vi "AlliGator Init Image Profile Window Menu.vi"(8 "error in":errorcluster, 11 "Menu in":refnum<k9>) -> (0 "error out":errorcluster)   [LabVIEW 2021, in "AlliGator Image Profile Window.lvlib"]
doc: "Initialize Profile Window menu."
uses:
  AlliGator Image Profile Window.lvlib
  Globals, Variables, Constants/AlliGator Variables List.ctl
  Image/Box Profile Type.ctl
  AlliGator Image Profile Intensity Type.ctl
  AlliGator Image Profile Average Intensity Type.ctl
  Globals, Variables, Constants/AlliGator Globals, Variables & Constants.lvlib
  Image/Image.lvlib
panel:
  # "see the AlliGator License on the block diagram (Ctrl+E or Window:Show Block Diagram)"
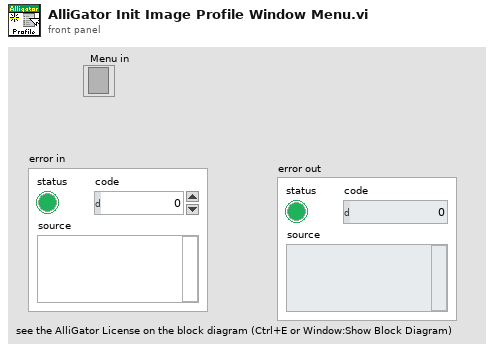
[diagram p1: front panel]
types:
  T1 = typedef "AlliGator Image Profile Window.lvlib/AlliGator Image Profile Average Intensity Type.ctl" = enum16{"Integrated Intensity", "Average Intensity", "Intensity-weighted Average Intensity"}
  T2 = typedef "AlliGator Image Profile Window.lvlib/AlliGator Image Profile Intensity Type.ctl" = enum16{"Raw Data", "Displayed Image", "Background-subtracted"}
  T3 = typedef "AlliGator Globals, Variables & Constants.lvlib/AlliGator Variables List.ctl" = enum16{"---- GUI ----", "GUI:Initialization Status", "GUI:State Indicators Refnum", "GUI:Original AlliGator Menu Items", "GUI:Current Action Loop State", "GUI:Script in progress", "GUI:Playback", "GUI:Loop Playback", "GUI:Search ROI Used", "GUI:Search ROI", "Decay Graph Max Legend Size", "Intensity Graph Max Legend Size", "Decay Statistics Graph Max Legend Size", "Phasor Graph Max Legend Size", "Phasor Ratio Graph Max Legend Size", "Lifetime Graph Max Legend Size", "---- Files ----", "Files:Export Dataset Frames as Individual Files", "Files:Show Batch Export Help Balloons", "Files:Frames in Dataset", "Files:ptu File Frame Start Indices", "Files:Current Frame in Dataset", "Files:Current Frame Timestamp", "Files:Dataset Loaded", "Files:Dataset Metadata", "Files:Dataset Channel", "Files:Dataset Data Description", "Files:Background Dataset Metadata", "Files:Background Dataset Channel", "Files:Background Dataset Data Description", "Files:Background File Subtraction", "Files:Background File Path", "Files:Background File Pile-up Correction", "Files:Background File Pixel Well Capacity", "Files:Background File Scaling Factor", "Files:Current Dataset Load Settings", "Files:Dataset Path", "Files:ICCD-specific Information", "Files:Macrotime Gate Separation", "------ Python Plugins ------", "Python Plugins:Information", "Python Plugins:Python Session", "Python Plugins:Valid Python Session?", "---- Source Image ----", "Source Image:ROIs", "Source Image:Current ROI", "Source Image:ROI Event Refnum", "X_Source Image Display Range", "X_Source Image Palette Information", "X_Type of Displayed Image", "X_Time Gate Slider", "Source Image:Palette List", "Source Image:Scale", "Source Image:ROI Overlay Color", "Source Image:Overlay to Erase", "Source Image:Is Displayed Image Accumulated", "Source Image:White Light Image Modified", "Source Image:Mask Image Modified", "---- Image Profile Window ----", "Image Profile:Window Event Refnum", "Image Profile:IntensityType", "Image Profile:Intensity Average Type", "Image Profile:Intensity-weighted SDV", "Image Profile:Box Profile Type", "Image Profile:Window Open", "Image Profile:Plotted Fit Parameter", "------ Phasor Graph -------", "Phasor Graph:Show Line", "---- Phasor Plot ---", "Phasor Plot:Parameters Changed", "Phasor Plot:FLI Dataset Modified since last Calculation", "Phasor Harmonics Data", "Selected Phasor Harmonics", "Phasor Harmonic Manager Event Refnum", "Phasor Plot:ROIs", "Phasor Plot:Current ROI", "Phasor Plot:ROI Event Refnum", "Phasor Plot:Image Reference Points", "Phasor Plot:Computed", "Phasor Plot:Palette Information", "Phasor Plot:Palette List", "Phasor Plot:Phasor Ratio Palette Information", "Phasor Plot:Phasor Ratio Palette List", "Phasor Plot:Image Scale", "Phasor Plot:Image Overlay to Erase", "Phasor Plot:Image Elements to Update", "Phasor Plot:Current Calculation Parameters", "Phasor Plot:Current Calibration Options", "Phasor Plot:Reset Cumulated Phasor Plot", "Phasor Plot:Reference 1", "Phasor Plot:Lifetime Reference 1", "Phasor Plot:Reference 1 Frequency", "Phasor Plot:Reference 2", "Phasor Plot:Lifetime Reference 2", "Phasor Plot:Reference 2 Frequency", "---- Decay Analysis ----", "Number of Selected Decays to Fit", "LS Fit Results", "LAR Fit Results", "BS Fit Results", "Last Decay Max - Min", "Best Fit Parameters", "Best Fit Parameter Names", "Actual Size X", "Actual Size Y", "Binning X", "Binning Y", "Actual # Gates", "Dataset Number", "Gates to...", "Gates Skipped", "Gates to keep", "Gate Step", "Gate Separation", "Reversed Gates", "Pile-up Correction", "Pixel Well Capacity", "Background Subtracted", "Background Subtraction Method", "Background Definition Range", "Background File (deprecated)", "Number of Dataset Accumulated", "Array of Accumulated Dataset Paths", "Do Averaged Datasets", "Destination File Path", "Process Plot Target", "Use 1/D as Phasor Frequency", "---- Decay Fit Parameter Map -----", "Decay Fit Parameter Map:Palette Information", "Decay Fit Parameter Map:Palette List", "---- Parameter Map ----", "Parameter Map:Palette Information", "Parameter Map:Palette List", "------- Local Decay Window ---------", "Local Decay Graph Window:Event Refnum", "Local Decay Graph Window:Use normalized IRF for convolution", "----- Miscellaneous ----", "Misc:Skippable Dialog Windows Status"}
  T4 = typedef "Image.lvlib/Box Profile Type.ctl" = enum16{"Full Width", "Half Width"}
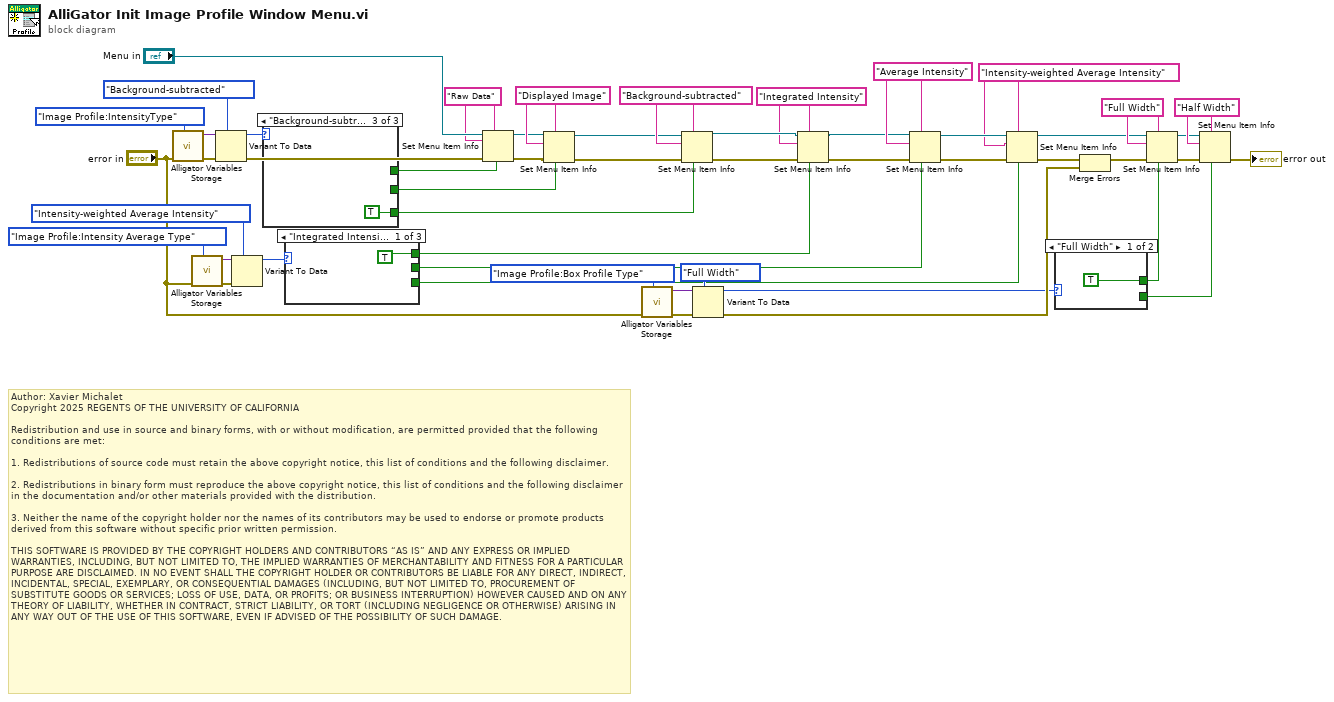
[diagram p0: block diagram]
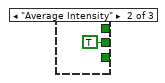
[diagram p2: hidden frame]
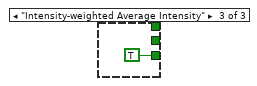
[diagram p3: hidden frame]
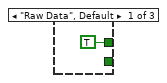
[diagram p4: hidden frame]
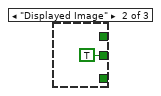
[diagram p5: hidden frame]
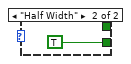
[diagram p6: hidden frame]
diagram:
  w3 = "Integrated Intensity" ("item tag")
  w14 = "Intensity-weighted Average Intensity" ("ItemTag")
  w15 = "Average Intensity" ("ItemTag")
  w47 = "Half Width" ("item tag")
  w46 = "Full Width" ("item tag")
  w42 = "Background-subtracted" ("ItemTag")
  w32 = "Raw Data" ("ItemTag")
  w33 = "Displayed Image" ("ItemTag")
  # "Author: Xavier Michalet\nCopyright 2025 REGENTS OF THE UNIVERSITY OF CALIFORNIA\n\nRedistribution and use in source and binary forms, with or without modification, are permitted provided that the following conditions are met:\n\n1. Redistributions of source code must retain the above copyright notice, this list of conditions and the following disclaimer.\n\n2. Redistributions in binary form must reproduce the above copyright notice, this list of conditions and the following disclaimer in the documentation and/or other materials provided with the distribution.\n\n3. Neither the name of the copyright holder nor the names of its contributors may be used to endorse or promote products derived from this software without specific prior written permission.\n\nTHIS SOFTWARE IS PROVIDED BY THE COPYRIGHT HOLDERS AND CONTRIBUTORS “AS IS” AND ANY EXPRESS OR IMPLIED WARRANTIES, INCLUDING, BUT NOT LIMITED TO, THE IMPLIED WARRANTIES OF MERCHANTABILITY AND FITNESS FOR A PARTICULAR PURPOSE ARE DISCLAIMED. IN NO EVENT SHALL THE COPYRIGHT HOLDER OR CONTRIBUTORS BE LIABLE FOR ANY DIRECT, INDIRECT, INCIDENTAL, SPECIAL, EXEMPLARY, OR CONSEQUENTIAL DAMAGES (INCLUDING, BUT NOT LIMITED TO, PROCUREMENT OF SUBSTITUTE GOODS OR SERVICES; LOSS OF USE, DATA, OR PROFITS; OR BUSINESS INTERRUPTION) HOWEVER CAUSED AND ON ANY THEORY OF LIABILITY, WHETHER IN CONTRACT, STRICT LIABILITY, OR TORT (INCLUDING NEGLIGENCE OR OTHERWISE) ARISING IN ANY WAY OUT OF THE USE OF THIS SOFTWARE, EVEN IF ADVISED OF THE POSSIBILITY OF SUCH DAMAGE."
  n1 = call "Alligator Variables Storage.vi"("AlliGator Variable"=AlliGator_Variables_List."Image Profile:IntensityType" ("Alligator Variable"), "Error In"="error in") -> ("Error Out"=w30:errorcluster, "Data out"=w25:variant)  [unwired: 7 in, 1 out]
  n2 = call "Alligator Variables Storage.vi"("AlliGator Variable"=AlliGator_Variables_List."Image Profile:Intensity Average Type" ("Alligator Variable"), "Error In"="error in") -> ("Error Out"=w12:errorcluster, "Data out"=w13:variant)  [unwired: 7 in, 1 out]
  n3 = Variant To Data(error in=w30, type=AlliGator_Image_Profile_Intensity_Type."Background-subtracted" ("Image Profile Intensity Type"), Variant=w25) -> (data=w23:T2, error out=w26:errorcluster)
  n4 = Variant To Data(error in=w12, type=AlliGator_Image_Profile_Average_Intensity_Type."Intensity-weighted Average Intensity" ("Image Profile Average Intenisty Type"), Variant=w13) -> (data=w11:T1)  [unwired: 1 out]
  n5 = case shown="\"Background-subtracted\"" w23 {
    tunnel: [TRUE ("checked") _ _] -> w22
    tunnel: [_ TRUE ("checked") _] -> w21
    tunnel: [_ _ TRUE ("checked")] -> w20
    frame "Raw Data", Default {
    }
    frame "Displayed Image" {
    }
    frame "Background-subtracted" {
    }
  }
  n6 = case shown="\"Integrated Intensity\", Default" w11 {
    tunnel: [_ TRUE ("checked") _] -> w9
    tunnel: [_ _ TRUE ("checked")] -> w8
    tunnel: [TRUE ("checked") _ _] -> w2
    frame "Integrated Intensity", Default {
    }
    frame "Average Intensity" {
    }
    frame "Intensity-weighted Average Intensity" {
    }
  }
  n7 = Set Menu Item Info(6:w22, 7:w32, 8:w26, 10:w32, 11:"Menu in") -> (0:w28:errorcluster, 3:w27:refnum<k9>)  [unwired: 2 in]
  n8 = Set Menu Item Info(6:w21, 7:w33, 8:w28, 10:w33, 11:w27) -> (0:w39:errorcluster, 3:w40:refnum<k9>)  [unwired: 2 in]
  n9 = call "Alligator Variables Storage.vi"("AlliGator Variable"=AlliGator_Variables_List."Image Profile:Box Profile Type" ("Alligator Variable"), "Error In"="error in") -> ("Error Out"=w36:errorcluster, "Data out"=w35:variant)  [unwired: 7 in, 1 out]
  n10 = Set Menu Item Info(6:w20, 7:w42, 8:w39, 10:w42, 11:w40) -> (0:w5:errorcluster, 3:w7:refnum<k9>)  [unwired: 2 in]
  n11 = Variant To Data(error in=w36, type=Box_Profile_Type."Full Width", Variant=w35) -> (data=w49:T4, error out=w51:errorcluster)
  n12 = Set Menu Item Info(6:w2, 7:w3, 8:w5, 10:w3, 11:w7) -> (0:w4:errorcluster, 3:w6:refnum<k9>)  [unwired: 2 in]
  n13 = Set Menu Item Info(6:w9, 7:w15, 8:w4, 10:w15, 11:w6) -> (0:w18:errorcluster, 3:w19:refnum<k9>)  [unwired: 2 in]
  n14 = Set Menu Item Info(6:w8, 7:w14, 8:w18, 10:w14, 11:w19) -> (0:w16:errorcluster, 3:w17:refnum<k9>)  [unwired: 2 in]
  n15 = case shown="\"Full Width\"" w49 {
    tunnel: [TRUE ("checked") _] -> w43
    tunnel: [_ TRUE ("checked")] -> w45
    frame "Full Width" {
    }
    frame "Half Width" {
    }
  }
  n16 = Merge Errors(w16, w51) -> (w50:errorcluster)
  n17 = Set Menu Item Info(6:w43, 7:w46, 8:w50, 10:w46, 11:w17) -> (0:w48:errorcluster, 3:w44:refnum<k9>)  [unwired: 2 in]
  n18 = Set Menu Item Info(6:w45, 7:w47, 8:w48, 10:w47, 11:w44) -> (0:→"error out":errorcluster)  [unwired: 2 in, 1 out]
